vi "Event handler-Restart.vi"(11 "Queue in":refnum<queue>) -> (0 "error out":errorcluster)   [LabVIEW 2020]
uses:
  Queue/Message Queue/Typedefs/Message Cluster.ctl
  Global Variables/General Globals.vi
panel:
  in  "Front Panel Window:Transparency %":u8=5
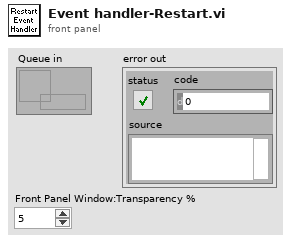
[diagram p1: front panel]
types:
  T1 = enum32{"Invalid", "Standard", "Closed", "Hidden", "Minimized", "Maximized"}
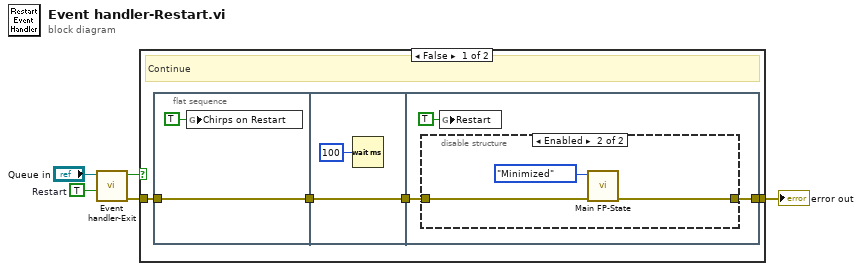
[diagram p0: block diagram]
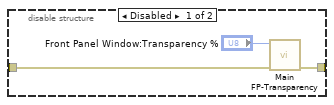
[diagram p2: hidden frame]
diagram:
  w5 = TRUE  # Restart
  n1 = call "Event handler-Exit.vi"("Restart (F)"=w5, "UI queue"="Queue in") -> ("error out"=w1:errorcluster, "Cancelled"=w4:bool)  [unwired: 8 in]
  n2 = case shown="False" w4 {
    tunnel: [w9 w23] -> w2
    tunnel: w1 -> [w8 w23]
    frame False {
      # "Continue"
      n3 = flat-sequence {
        tunnel: w8 -> [w11]
        tunnel: [w11] -> w7
        tunnel: w7 -> [w13]
        tunnel: [w13] -> w6
        tunnel: [w16] -> w9
        tunnel: w6 -> [w15]
        frame #0 {
          n4 = global write "General Globals.vi" "Chirps on Restart"(TRUE ("Restart")) -> ()
        }
        frame #1 {
          n5 = Wait (ms)(milliseconds to wait=u32 100) -> ()  [unwired: 1 out]
        }
        frame #2 {
          n6 = disable-structure shown="Enabled" {
            disable-tunnel: [w19 w20] -> w16
            disable-tunnel: w15 -> [w18 w21]
            frame Disabled {
              n7 = call "Main FP-Transparency.vi"("error in (no error)"=w18, "Front Panel Window:Transparency"="Front Panel Window:Transparency %") -> ("error out"=w19:errorcluster)  [unwired: 9 in]
            }
            frame Enabled {
              n8 = call "Main FP-State.vi"("error in (no error)"=w21, "Front Panel Window:State"=T1."Minimized") -> ("error out"=w20:errorcluster)  [unwired: 9 in]
            }
          }
          n9 = global write "General Globals.vi" "Restart"(TRUE ("Restart")) -> ()
        }
      }
    }
    frame True {
      # "Cancelled"
    }
  }
  "error out" <- w2
